vi "LINC Connect.vi"(6 "port config":T1[](array[typedef]), 7 "timeout ms (1000)":i32=1000, 8 "error in (no error)":errorcluster, 9 "ports":u16[](array[numeric]), 10 "address":string="localhost", 11 "LINC session":refnum<class "LINC.lvclass">) -> (0 "error out":errorcluster, 3 "dup LINC session":refnum<class "LINC.lvclass">)   [LabVIEW 2018, in "STEPkgDriver_LINC.lvlib" / "LINC.lvclass"]
uses:
  LINC.lvclass
  LINC Global Session Mode.ctl
  STEPkgDriver_LINC.lvlib
  LINC Global Config Mode.ctl
  LINC Config.ctl
  LINC Port Config.ctl
panel:
  in  "Hidden":bool
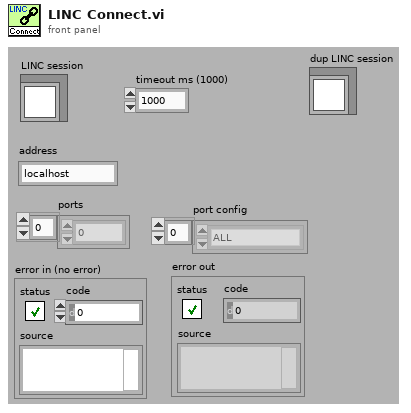
[diagram p1: front panel]
types:
  T1 = typedef "STEPkgDriver_LINC.lvlib/LINC Port Config.ctl" = enum16{"ALL", "CMD_ALL", "TLM_ALL", "TLM_BASIC"}
  T2 = typedef "STEPkgDriver_LINC.lvlib/LINC Config.ctl" = cluster{"cmd callback":refnum<vi>, "tlm callback":refnum<vi>, "cmd ID bitoffset":i32, "cmd ID bitsize":i32, "cmd IDs":i32[], "tlm ID bitoffset":i32, "tlm ID bitsize":i32, "tlm IDs":i32[], "cmd header fields":i32, "tlm header fields":i32, "tlm header size":i32}
  T3 = typedef "STEPkgDriver_LINC.lvlib/LINC Global Config Mode.ctl" = enum16{"INIT", "CLEAR", "SET_CMD_CB", "SET_TLM_CB", "SET_CMD_FIELDS", "SET_TLM_FIELDS", "SET_ID", "GET_CONFIG"}
  T4 = typedef "STEPkgDriver_LINC.lvlib/LINC Global Session Mode.ctl" = enum16{"INIT", "CLEAR", "ADD_SESSION", "SET_CONNECTION", "SET_LISTENER", "SET_REFERENCE", "GET_SESSION"}
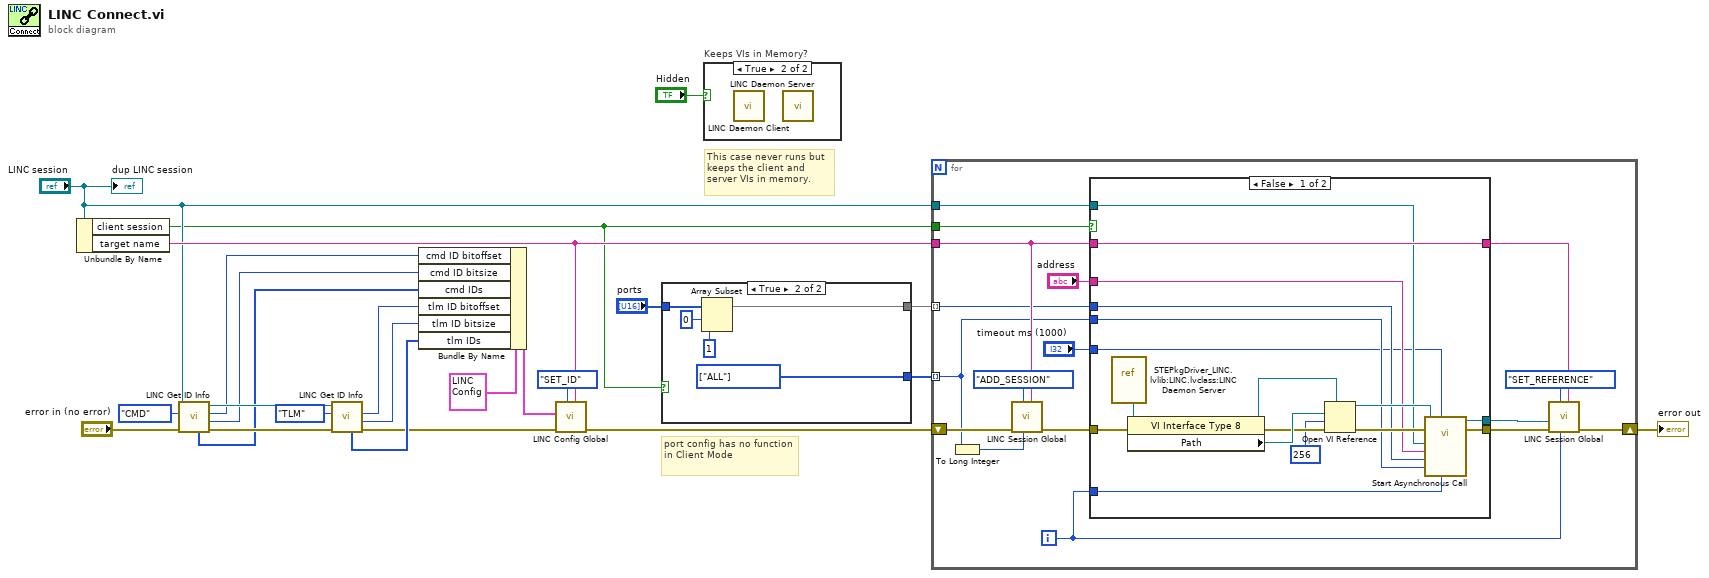
[diagram p0: block diagram]
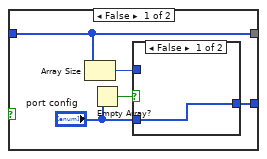
[diagram p3: hidden frame]
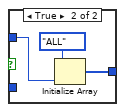
[diagram p4: hidden frame]
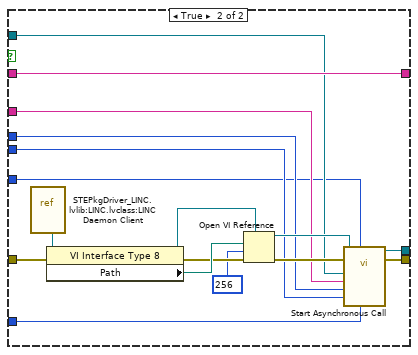
[diagram p5: hidden frame]
diagram:
  # "port config has no function in Client Mode"
  # "This case never runs but\nkeeps the client and\nserver VIs in memory."
  n1 = Unbundle By Name("LINC session") -> ("client session"=w1:bool, "target name"=w5:string)
  n2 = call "LINC Get ID Info.vi"("error in (no error)"="error in (no error)", "mode (CMD)"=enum16{"CMD", "TLM"}."CMD", "LINC session"="LINC session") -> ("error out"=w18:errorcluster, "bit size"=w15:i32, "bit offset"=w16:i32, "dup LINC session"=w17:refnum<class "LINC.lvclass">, "IDs"=w14:i32[])  [unwired: 4 in]
  n3 = call "LINC Get ID Info.vi"("error in (no error)"=w18, "mode (CMD)"=enum16{"CMD", "TLM"}."TLM", "LINC session"=w17) -> ("error out"=w9:errorcluster, "bit size"=w12:i32, "bit offset"=w13:i32, "IDs"=w11:i32[])  [unwired: 4 in, 1 out]
  n4 = Bundle By Name(cluster=T2 {"cmd callback"=refnum, "tlm callback"=refnum, "cmd ID bitoffset"=0, "cmd ID bitsize"=0, "cmd IDs"=[], "tlm ID bitoffset"=0, "tlm ID bitsize"=0, "tlm IDs"=[], "cmd header fields"=0, "tlm header fields"=0, "tlm header size"=0} ("config in"), "cmd ID bitoffset"=w16, "cmd ID bitsize"=w15, "cmd IDs"=w14, "tlm ID bitoffset"=w13, "tlm ID bitsize"=w12, "tlm IDs"=w11) -> (w21:T2)
  n5 = call "LINC Config Global.vi"("target name"=w5, "mode"=LINC_Global_Config_Mode."SET_ID", "error in (no error)"=w9, "config in"=w21) -> ("error out"=w6:errorcluster)  [unwired: 6 in, 1 out]
  n6 = case shown="True" w1 {
    tunnel: "ports" -> [w26 w38]
    tunnel: [w26 w37] -> w23
    tunnel: [w27 w34] -> w2
    frame False {
      n7 = Array Size(array=w26) -> (size(s)=w25:i32)
      n8 = Empty Array?(array="port config") -> (empty?=w29:bool)
      n9 = case shown="False" w29 {
        tunnel: "port config" -> [w30 _]
        tunnel: [w30 w32] -> w27
        tunnel: w25 -> [_ w33]
        frame False {
        }
        frame True {
          n10 = Initialize Array(LINC_Port_Config."ALL" ("port config"), w33) -> (w32:T1[])
        }
      }
    }
    frame True {
      w34 = T1[] [enum."ALL"] items=["ALL", "CMD_ALL", "TLM_ALL", "TLM_BASIC"] ("port config")
      n11 = Array Subset(array=w38, index=0, length=1) -> (w37:u16[])
    }
  }
  n12 = case "Keeps VIs in Memory?" shown="True" "Hidden" {
    frame False {
    }
    frame True {
      n13 = call "LINC Daemon Client.vi"() -> ()  [unwired: 12 in]
      n14 = call "LINC Daemon Server.vi"() -> ()  [unwired: 12 in]
    }
  }
  n15 = for {
    shift-right: [w52] -> w22
    shift-left: w6 -> [w55]
    tunnel: w23 -> [w44] mode=indexing
    tunnel: w5 -> [w46]
    tunnel: "LINC session" -> [w47]
    tunnel: w2 -> [w42] mode=indexing
    tunnel: w1 -> [w49]
    i -> [w43]
    n16 = To Long Integer(number=w42) -> (32bit integer=w51:i32)
    n17 = call "LINC Session Global.vi"("target name"=w46, "value in"=w51, "mode"=LINC_Global_Session_Mode."ADD_SESSION", "error in (no error)"=w55) -> ("error out"=w50:errorcluster)  [unwired: 3 in, 4 out]
    n18 = case shown="False" w49 {
      tunnel: w50 -> [w65 w82]
      tunnel: [w62 w79] -> w48
      tunnel: w47 -> [w61 w78]
      tunnel: w46 -> [w64 w81]
      tunnel: [w64 w81] -> w45
      tunnel: w44 -> [w59 w76]
      tunnel: w43 -> [w57 w74]
      tunnel: w42 -> [w58 w75]
      tunnel: [w63 w80] -> w41
      tunnel: "timeout ms (1000)" -> [w56 w73]
      tunnel: "address" -> [w60 w77]
      frame False {
        n19 = vi-ref "STEPkgDriver_LINC.lvlib:LINC.lvclass:LINC Daemon Server.vi"() -> (w72:refnum<vi>)
        n20 = property class="VI Interface Type 8"(reference=w72, error in=w65) -> (reference out=w71:refnum<vi>, error out=w69:errorcluster, "Path"=w70:path)
        n21 = Open VI Reference(type specifier VI Refnum (for type only)=w71, vi path=w70, options=256, error in (no error)=w69) -> (vi reference=w68:refnum<vi>, error out=w67:errorcluster)  [unwired: 2 in]
        n22 = call-by-ref "Start Asynchronous Call"(reference=w68, error in=w67, "instance"=w57, "timeout ms (1000)"=w56, "port config"=w58, "port"=w59, "address"=w60, "LINC session"=w61) -> (reference out=w63:refnum<vi>, error out=w62:errorcluster)  [unwired: 6 in]
      }
      frame True {
        n23 = vi-ref "STEPkgDriver_LINC.lvlib:LINC.lvclass:LINC Daemon Client.vi"() -> (w89:refnum<vi>)
        n24 = property class="VI Interface Type 8"(reference=w89, error in=w82) -> (reference out=w88:refnum<vi>, error out=w86:errorcluster, "Path"=w87:path)
        n25 = Open VI Reference(type specifier VI Refnum (for type only)=w88, vi path=w87, options=256, error in (no error)=w86) -> (vi reference=w85:refnum<vi>, error out=w84:errorcluster)  [unwired: 2 in]
        n26 = call-by-ref "Start Asynchronous Call"(reference=w85, error in=w84, "instance"=w74, "timeout ms (1000)"=w73, "port config"=w75, "port"=w76, "address"=w77, "LINC session"=w78) -> (reference out=w80:refnum<vi>, error out=w79:errorcluster)  [unwired: 6 in]
      }
    }
    n27 = call "LINC Session Global.vi"("target name"=w45, "value in"=w43, "mode"=LINC_Global_Session_Mode."SET_REFERENCE", "error in (no error)"=w48, "reference in"=w41) -> ("error out"=w52:errorcluster)  [unwired: 2 in, 4 out]
  }
  "error out" <- w22
  "dup LINC session" <- "LINC session"
